vi "re_obj_Datalog Database Info.vi"(0 "method":T9, 1 "initial number (NaN)":dbl=nan format="%.2f", 2 "database {initialize}":path, 5 "tag or base tag":string, 7 "tag config in":T4 {"logging parameters" format="%.2e"; "precision" items=["0", "1", "2", "3", "4", "5", "6", "7", "8", "9", "10", "11", "12", "13", "14", "15", "16", "17"]; "limit delay" format="%.2e"; "deadband" format="%.2e"}, 9 "subsets in":T1[](array[typedef]), 11 "tag index/change#":i32, 12 "meta specifier (not a meta)":T3=enum."not a meta", 13 "initial string (\"\")":string) -> (3 "mode":T2, 4 "tag config list":T4[](array[typedef]) {"logging parameters" format="%.2e"; "precision" items=["0", "1", "2", "3", "4", "5", "6", "7", "8", "9", "10", "11", "12", "13", "14", "15", "16", "17"]; "limit delay" format="%.2e"; "deadband" format="%.2e"}, 6 "#tags/change#":i32, 8 "tag config out":T4 {"logging parameters" format="%.2e"; "precision" items=["0", "1", "2", "3", "4", "5", "6", "7", "8", "9", "10", "11", "12", "13", "14", "15", "16", "17"]; "limit delay" format="%.2e"; "deadband" format="%.2e"}, 10 "subsets out":T1[](array[typedef]), 14 "path":path, 15 "error out":errorcluster)   [LabVIEW 2012]
doc: "Instantiatable object that represents a database through a list of tags and other information. It provides and in-memory copy of the tag info files contained in the tag log directories. These directories are located under the configured data base path.\n\nWhich methods are allowed depends on the mode of the database. When \"locked\" no changes are allowed. When \"unlocked\" everything is allowed. When \"live\" a subset of changes is allowed consistent with ongoing logging.\n\nThe order of the list is kept sorted by tag name. The info cluster holds a seemingly redundant tag index. Its purpose is to allow a list exported via {get list} to be resorted by some other criterion without loosing track of the index.\n\nNote that the handling of the various tag info elements differs. Some are set only when the tag log is first created, some can be set only when the tag is configured before data logging starts, some are determined programatically, and others are modifyable at any time."
uses:
  typedefs/t_DataLog Tag Info List Methods.ctl
  typedefs/t_Datalog Datebase Modes.ctl
  typedefs/clusters/t_DataLog Tag Config.ctl
  typedefs/t_DataLog Temporal Types.ctl
  typedefs/t_DataLog Value Types.ctl
  typedefs/t_DataLog Numerical Format.ctl
  typedefs/t_DataLog Logging Algorithms.ctl
  typedefs/clusters/t_DataLog Tag Subset.ctl
  typedefs/et_DataLog Meta Tag Specifier.ctl
  typedefs/t_Datalog Subsets Actions.ctl
  typedefs/t_DataLog Expression Update Timing Methods.ctl
  subvis/private/glb_DataLog Runtime Parameterisation.vi
  subvis/private/glb_DataLog MCVD.vi
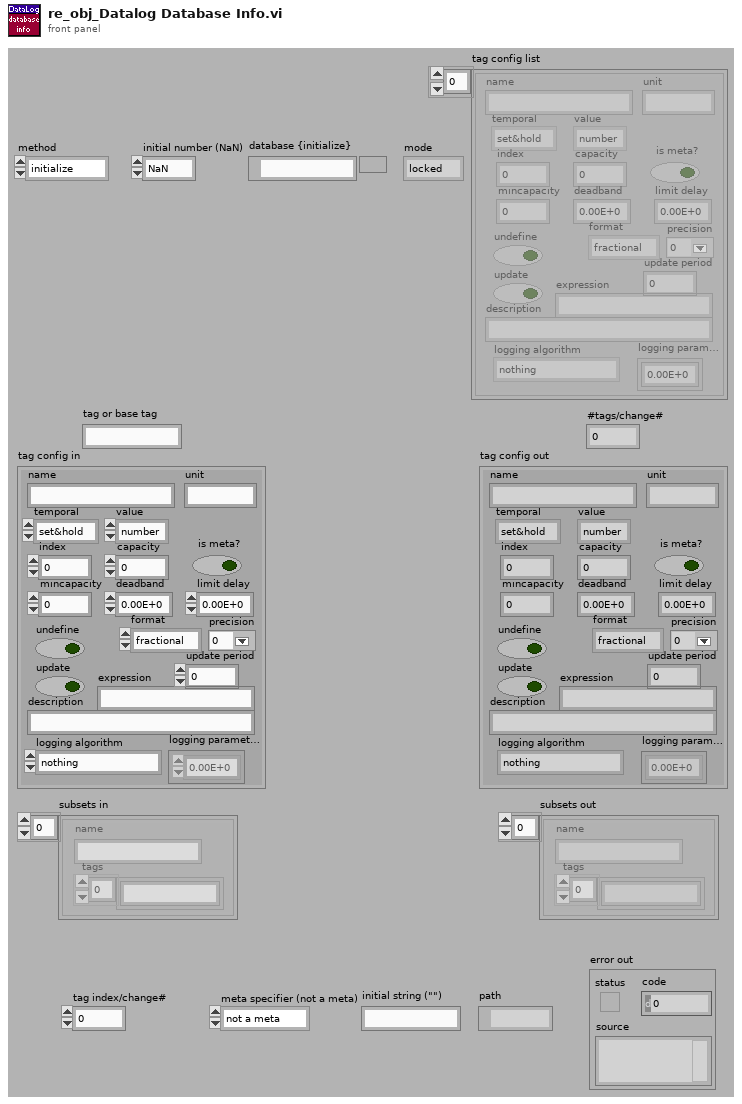
[diagram p1: front panel]
types:
  T1 = typedef "t_DataLog Tag Subset.ctl" = cluster{"name":string, "tags":string[]}
  T2 = typedef "t_Datalog Datebase Modes.ctl" = enum16{"locked", "unlocked", "live", "mirrored"}
  T3 = typedef "et_DataLog Meta Tag Specifier.ctl" = enum32{"warn_lo", "warn_hi", "A_lo", "A_hi", "B_lo", "B_hi", "C_lo", "C_hi", "D_lo", "D_hi", "E_lo", "E_hi", "F_lo", "F_hi", "G_lo", "G_hi", "H_lo", "H_hi", "I_lo", "I_hi", "J_lo", "J_hi", "K_lo", "K_hi", "L_lo", "L_hi", "M_lo", "M_hi", "N_lo", "N_hi", "min", "max", "not a meta"}
  T4 = typedef "t_DataLog Tag Config.ctl" = cluster{"name":string, "unit":string, "temporal":T5, "value":T6, "index":i32, "capacity":i32, "is meta?":bool, "mincapacity":i32, "deadband":dbl, "limit delay":dbl, "format":T7, "precision":u8, "undefine":bool, "update":bool, "update period":u16, "expression":string, "description":string, "logging algorithm":T8, "logging parameters":dbl[]}
  T5 = typedef "t_DataLog Temporal Types.ctl" = enum16{"set&hold", "sample", "event"}
  T6 = typedef "t_DataLog Value Types.ctl" = enum16{"number", "string"}
  T7 = typedef "t_DataLog Numerical Format.ctl" = enum8{"fractional", "exponential", "engineering"}
  T8 = typedef "t_DataLog Logging Algorithms.ctl" = enum16{"nothing", "changes", "everything", "every Nth", "time threshold", "value threshold + prior", "t or v threshold", "t or v threshold + prior"}
  T9 = typedef "t_DataLog Tag Info List Methods.ctl" = enum16{"initialize", "create", "create empty", "rename", "delete", "test tag", "get", "get by name", "get default", "get list", "get path", "get subsets", "set subsets", "set config", "set capacity", "#tags", "go live", "set unlocked", "set mirrored"}
  T10 = typedef "t_Datalog Subsets Actions.ctl" = enum16{"load", "rename", "delete", "save"}
  T11 = typedef "t_DataLog Expression Update Timing Methods.ctl" = enum16{"initialize", "schedule", "make due", "next due", "cleanup"}
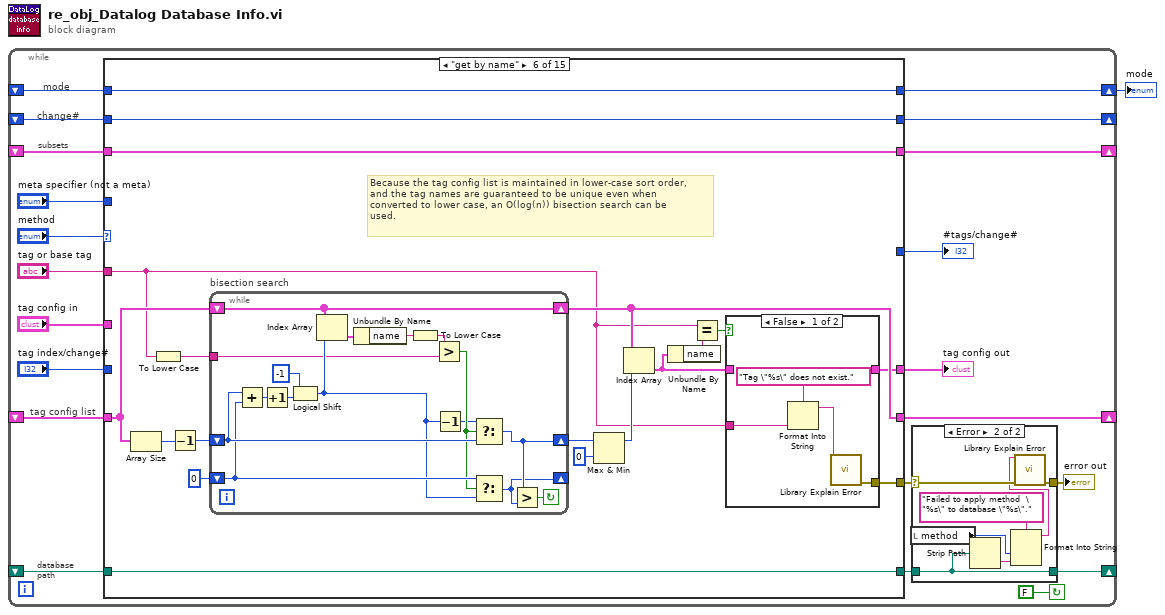
[diagram p0: block diagram]
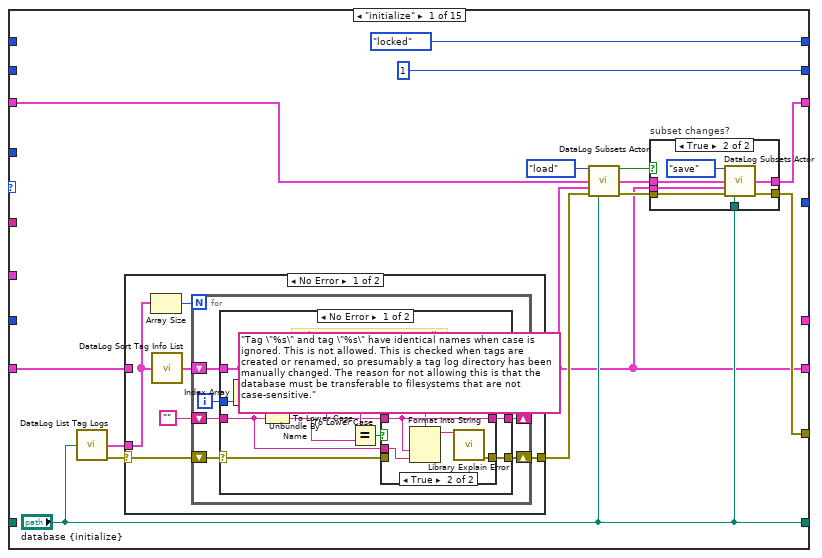
[diagram p3: hidden frame]
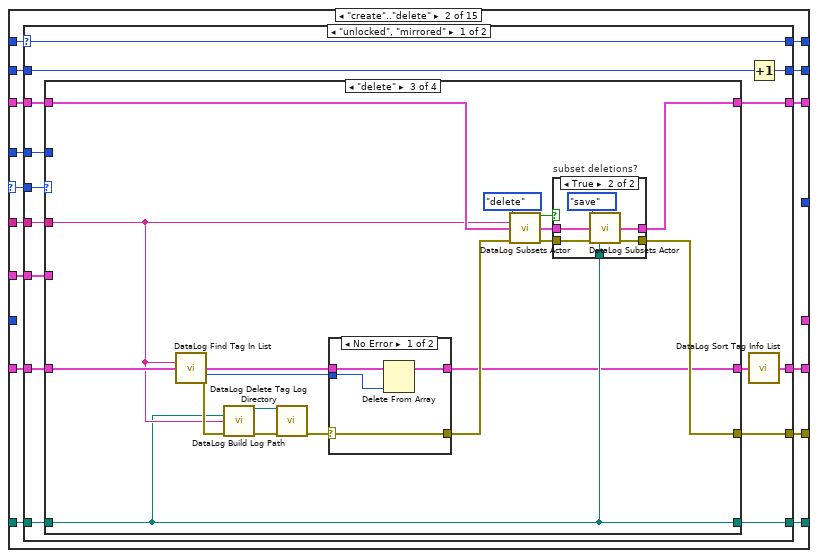
[diagram p8: hidden frame]
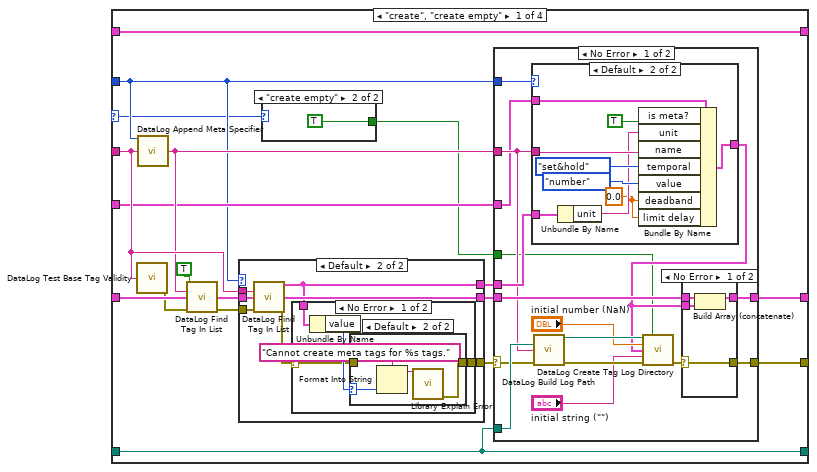
[diagram p9: hidden frame]
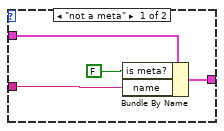
[diagram p11: hidden frame]
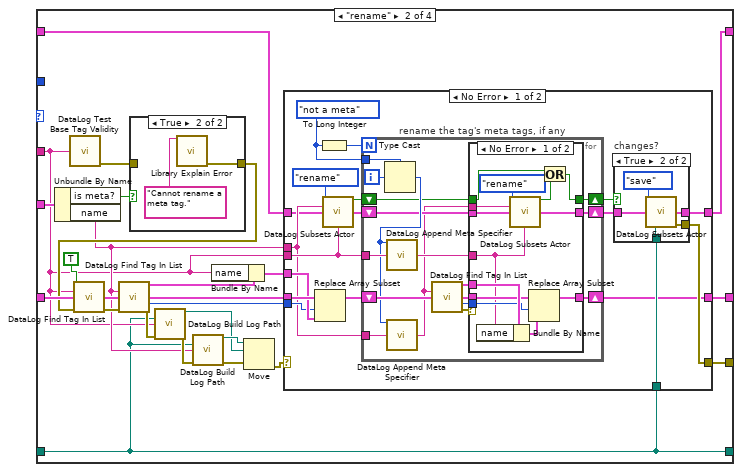
[diagram p17: hidden frame]
diagram:
  n1 = while {
    shift-right: [w21] -> _
    shift-left: _ -> [w20]
    shift-right: [w8] -> w1
    shift-left: _ -> [w18]
    shift-right: [w12] -> _
    shift-left: _ -> [w15]
    shift-right: [w5] -> _
    shift-left: _ -> [w6]
    shift-right: [w3] -> _
    shift-left: _ -> [w4]
    stop <- FALSE continue-if-true
    # "change#"
    # "subsets"
    # "database\npath"
    # "mode"
    # "tag config list"
    n2 = case shown="\"get by name\"" "method" {
      selector: "method" -> [_ w105 w341 _ _ _ _ _ _ _ w465 _ _ _ _]
      tunnel: w20 -> [w44 w104 w340 w364 w373 w384 w421 w439 w454 w458 w473 w589 w595 w601 w607]
      tunnel: [w36 w102 w338 w363 w373 w381 w420 w438 w454 w458 w470 w587 w595 w601 w607] -> w21
      tunnel: "tag config in" -> [_ w101 w337 _ _ _ _ _ _ _ w472 w585 _ _ _]
      tunnel: w18 -> [_ w107 w343 w367 w374 w393 w425 w447 w453 w459 w467 w583 w594 w598 _]
      tunnel: [t_Datalog_Datebase_Modes."locked" ("mode") w106 w342 w367 w374 w393 w425 w447 w453 w459 w466 w583 w594 t_Datalog_Datebase_Modes."unlocked" ("mode") t_Datalog_Datebase_Modes."mirrored" ("mode")] -> w8
      tunnel: [w39 w103 w339 w362 _ w375 w419 _ _ _ w471 _ _ _ _] -> w14
      tunnel: "tag or base tag" -> [_ w100 w336 w361 _ w376 w422 _ _ _ w464 _ _ _ _]
      tunnel: w15 -> [_ w99 w335 w360 w372 w392 w424 w446 w452 w457 w469 w582 w593 w600 w606]
      tunnel: ["database {initialize}" w98 w334 w360 w372 w392 w424 w446 w452 w457 w468 w582 w593 w600 w606] -> w13
      tunnel: [_ _ _ _ w371 w378 w417 _ _ _ _ _ _ _ _] -> w11
      tunnel: "tag index/change#" -> [_ _ _ _ w370 _ _ w444 _ _ _ w581 _ _ _]
      tunnel: "meta specifier (not a meta)" -> [_ w97 w333 _ _ _ _ _ _ _ _ _ _ _ _]
      tunnel: [w34 w95 w331 w359 w369 w391 w416 w445 w451 w456 w462 w580 w592 w597 w604] -> w5
      tunnel: w6 -> [w41 w96 w332 w359 w369 w391 w416 w445 w451 w456 w463 w580 w592 w597 w604]
      tunnel: w4 -> [_ w94 w330 w358 w368 w390 w415 w440 w450 w455 w461 w579 w590 w596 w603]
      tunnel: [1 w93 w329 w358 w368 w390 w415 w440 w450 w455 w460 w578 w590 w596 w603] -> w3
      tunnel: [_ _ _ _ _ _ _ w440 _ _ _ _ w591 _ _] -> w2
      frame "initialize" {
        n3 = call "DataLog List Tag Logs.vi"("database path"="database {initialize}") -> ("tag info list"=w45:T4[], "error out"=w46:errorcluster)  [unwired: 13 in]
        n4 = case shown="No Error" w46 {
          selector: w46 -> [w61 w92]
          tunnel: [w60 w92] -> w40
          tunnel: [w59 w91] -> w36
          tunnel: w45 -> [w56 _]
          tunnel: w44 -> [_ w91]
          frame No Error {
            n5 = Array Size(array=w56) -> (size(s)=w57:i32)
            n6 = call "DataLog Sort Tag Info List.vi"("tag list in"=w56) -> ("tag list out"=w62:T4[])  [unwired: 14 in]
            n7 = for {
              N: w57 -> [_]
              shift-right: [w65] -> w60
              shift-left: w61 -> [w67]
              shift-right: [w66] -> w59
              shift-left: w62 -> [w69]
              shift-right: [w64] -> _
              shift-left: "" -> [w63]
              i -> [w68]
              n8 = case shown="No Error" w67 {
                selector: w67 -> [w74 w89]
                tunnel: w69 -> [w79 w90]
                tunnel: w68 -> [w80 _]
                tunnel: [w79 w90] -> w66
                tunnel: [w73 w89] -> w65
                tunnel: [w71 w88] -> w64
                tunnel: w63 -> [w70 w88]
                frame No Error {
                  # "Make sure tag names are still\ncase-independently unique."
                  n9 = Index Array(array=w79, index=w80) -> (element=w78:T4)
                  n10 = To Lower Case(string=w70) -> (all lower case string=w76:string)
                  n11 = Unbundle By Name(w78) -> ("name"=w72:string)
                  n12 = To Lower Case(string=w72) -> (all lower case string=w77:string)
                  n13 = Equal?(x=w77, y=w76) -> (x = y?=w75:bool)
                  n14 = case shown="True" w75 {
                    tunnel: w74 -> [w82 _]
                    tunnel: [w82 w87] -> w73
                    tunnel: w72 -> [w81 w85]
                    tunnel: [w81 w85] -> w71
                    tunnel: w70 -> [_ w84]
                    frame False {
                    }
                    frame True {
                      n15 = Format Into String(format string="Tag \"%s\" and tag \"%s\" have identical names when case is ignored. This is not allowed. This is checked when tags are created or renamed, so presumably a tag log directory has been manually changed. The reason for not allowing this is that the database must be transferable to filesystems that are not case-sensitive.", w85, w84) -> (resulting string=w86:string)  [unwired: 2 in, 1 out]
                      n16 = call "Library Explain Error.vi"("explanation prefix (none)"=w86) -> ("explained error"=w87:errorcluster)  [unwired: 14 in]
                    }
                  }
                }
                frame Error {
                }
              }
            }
          }
          frame Error {
          }
        }
        n17 = call "DataLog Subsets Actor.vi"("action"=t_Datalog_Subsets_Actions."load", "subsets in"=w41, "tag config list"=w36, "error in (no error)"=w40, "database path"="database {initialize}") -> ("changes"=w33:bool, "subset out"=w35:T1[], "error out"=w38:errorcluster)  [unwired: 8 in]
        n18 = case "subset changes?" shown="True" w33 {
          tunnel: [w47 w54] -> w39
          tunnel: w38 -> [w47 w53]
          tunnel: "database {initialize}" -> [_ w52]
          tunnel: w36 -> [_ w51]
          tunnel: w35 -> [w48 w50]
          tunnel: [w48 w49] -> w34
          frame False {
          }
          frame True {
            n19 = call "DataLog Subsets Actor.vi"("action"=t_Datalog_Subsets_Actions."save", "subsets in"=w50, "tag config list"=w51, "error in (no error)"=w53, "database path"=w52) -> ("subset out"=w49:T1[], "error out"=w54:errorcluster)  [unwired: 8 in, 1 out]
          }
        }
      }
      frame "create".."delete" {
        n20 = case shown="\"unlocked\", \"mirrored\"" w107 {
          selector: w107 -> [w109 w324]
          tunnel: [w109 w324] -> w106
          tunnel: w105 -> [w122 _]
          tunnel: w104 -> [w121 w325]
          tunnel: [w118 w328] -> w103
          tunnel: [w116 w325] -> w102
          tunnel: w101 -> [w119 _]
          tunnel: w100 -> [w120 _]
          tunnel: w99 -> [w115 w323]
          tunnel: [w113 w323] -> w98
          tunnel: w97 -> [w114 _]
          tunnel: w96 -> [w112 w322]
          tunnel: [w111 w322] -> w95
          tunnel: w94 -> [w110 w321]
          tunnel: [w108 w321] -> w93
          frame "unlocked", "mirrored" {
            n21 = case shown="\"delete\"" w122 {
              selector: w122 -> [w124 _ _ _]
              tunnel: w121 -> [w140 w209 w301 w320]
              tunnel: [w136 w204 w286 w320] -> w117
              tunnel: w120 -> [w134 w199 w294 _]
              tunnel: w119 -> [w129 w222 _ _]
              tunnel: [w137 w200 w289 _] -> w118
              tunnel: w115 -> [w126 w198 w287 w319]
              tunnel: w114 -> [w128 _ _ _]
              tunnel: [w126 w198 w287 w319] -> w113
              tunnel: w112 -> [w125 w203 w295 w318]
              tunnel: [w125 w202 w291 w318] -> w111
              frame "create", "create empty" {
                n22 = call "DataLog Test Base Tag Validity.vi"("base tag"=w134) -> ("error out"=w138:errorcluster)  [unwired: 13 in, 1 out]
                n23 = call "DataLog Append Meta Specifier.vi"("meta specifier"=w128, "tag in"=w134) -> ("tag out"=w130:string)  [unwired: 13 in]
                n24 = call "DataLog Find Tag In List.vi"("may not exist (false)"=TRUE, "tag"=w130, "tag config list in"=w140, "error in (no error)"=w138) -> ("tag config list out"=w131:T4[], "error out"=w135:errorcluster)  [unwired: 8 in, 2 out]
                n25 = case shown="Default" w128 {
                  tunnel: w135 -> [w179 w187]
                  tunnel: [w179 w181] -> w127
                  tunnel: w134 -> [_ w186]
                  tunnel: w131 -> [w180 w185]
                  tunnel: [w180 w184] -> w133
                  tunnel: [_ w183] -> w132
                  frame "not a meta" {
                  }
                  frame Default {
                    n26 = call "DataLog Find Tag In List.vi"("tag"=w186, "tag config list in"=w185, "error in (no error)"=w187) -> ("tag config out"=w183:T4, "tag config list out"=w184:T4[], "error out"=w182:errorcluster)  [unwired: 9 in, 1 out]
                    n27 = case shown="No Error" w182 {
                      selector: w182 -> [w189 w197]
                      tunnel: w183 -> [w191 _]
                      tunnel: [w188 w197] -> w181
                      frame No Error {
                        n28 = Unbundle By Name(w191) -> ("value"=w190:T6)
                        n29 = case shown="Default" w190 {
                          selector: w190 -> [_ w194]
                          tunnel: w189 -> [w192 _]
                          tunnel: [w192 w196] -> w188
                          frame "number" {
                          }
                          frame Default {
                            n30 = Format Into String(format string="Cannot create meta tags for %s tags.", w194) -> (resulting string=w195:string)  [unwired: 2 in, 1 out]
                            n31 = call "Library Explain Error.vi"("explanation prefix (none)"=w195) -> ("explained error"=w196:errorcluster)  [unwired: 14 in]
                          }
                        }
                      }
                      frame Error {
                      }
                    }
                  }
                }
                n32 = case shown="\"create empty\"" w124 {
                  tunnel: [_ TRUE] -> w123
                  frame Default {
                  }
                  frame "create empty" {
                  }
                }
                n33 = case shown="No Error" w127 {
                  selector: w127 -> [w144 w177]
                  tunnel: [w154 w177] -> w137
                  tunnel: [w153 w178] -> w136
                  tunnel: w133 -> [w151 w178]
                  tunnel: w132 -> [w150 _]
                  tunnel: w126 -> [w149 _]
                  tunnel: w130 -> [w147 _]
                  tunnel: w129 -> [w146 _]
                  tunnel: w128 -> [w145 _]
                  tunnel: w123 -> [w142 _]
                  frame No Error {
                    n34 = case shown="Default" w145 {
                      tunnel: w147 -> [w160 w170]
                      tunnel: w150 -> [_ w166]
                      tunnel: [w159 w164] -> w148
                      tunnel: w146 -> [w158 w163]
                      frame "not a meta" {
                        n35 = Bundle By Name(cluster=w158, "is meta?"=FALSE, "name"=w160) -> (w159:T4)
                      }
                      frame Default {
                        w162 = 0.0 ("deadband")
                        n36 = Unbundle By Name(w166) -> ("unit"=w165:string)
                        n37 = Bundle By Name(cluster=w163, "is meta?"=TRUE, "unit"=w165, "name"=w170, "temporal"=t_DataLog_Temporal_Types."set&hold", "value"=t_DataLog_Value_Types."number" ("valuation"), "deadband"=w162, "limit delay"=w162) -> (w164:T4)
                      }
                    }
                    n38 = call "DataLog Build Log Path.vi"("database path"=w149, "tag"=w147, "error in (no error)"=w144) -> ("tag log directory"=w156:path, "error out"=w157:errorcluster)  [unwired: 11 in]
                    n39 = call "DataLog Create Tag Log Directory.vi"("tag log directory"=w156, "no initial? (false)"=w142, "initial number (NaN)"="initial number (NaN)", "initial tag config"=w148, "initial string (\"\")"="initial string (\"\")", "error in (no error)"=w157) -> ("error out"=w155:errorcluster)  [unwired: 8 in, 1 out]
                    n40 = case shown="No Error" w155 {
                      selector: w155 -> [w171 w176]
                      tunnel: [w171 w176] -> w154
                      tunnel: [w173 w175] -> w153
                      tunnel: w151 -> [w174 w175]
                      tunnel: w148 -> [w172 _]
                      frame No Error {
                        n41 = Build Array (concatenate)(w174, w172) -> (w173:T4[])
                      }
                      frame Error {
                      }
                    }
                  }
                  frame Error {
                  }
                }
              }
              frame "rename" {
                n42 = Unbundle By Name(w222) -> ("is meta?"=w221:bool, "name"=w201:string)
                n43 = call "DataLog Test Base Tag Validity.vi"("base tag"=w199) -> ("error out"=w211:errorcluster)  [unwired: 13 in, 1 out]
                n44 = case shown="True" w221 {
                  tunnel: w211 -> [w283 _]
                  tunnel: [w283 w285] -> w206
                  frame False {
                  }
                  frame True {
                    n45 = call "Library Explain Error.vi"("explanation prefix (none)"="Cannot rename a meta tag.") -> ("explained error"=w285:errorcluster)  [unwired: 14 in]
                  }
                }
                n46 = call "DataLog Find Tag In List.vi"("may not exist (false)"=TRUE, "tag"=w199, "tag config list in"=w209, "error in (no error)"=w206) -> ("tag config list out"=w208:T4[], "error out"=w207:errorcluster)  [unwired: 8 in, 2 out]
                n47 = call "DataLog Find Tag In List.vi"("tag"=w201, "tag config list in"=w208, "error in (no error)"=w207) -> ("tag config out"=w212:T4, "tag config list out"=w213:T4[], "tag index"=w214:i32, "error out"=w210:errorcluster)  [unwired: 9 in]
                n48 = call "DataLog Build Log Path.vi"("database path"=w198, "tag"=w199, "error in (no error)"=w210) -> ("tag log directory"=w217:path, "error out"=w219:errorcluster)  [unwired: 11 in]
                n49 = call "DataLog Build Log Path.vi"("database path"=w198, "tag"=w201, "error in (no error)"=w219) -> ("tag log directory"=w220:path, "error out"=w218:errorcluster)  [unwired: 11 in]
                n50 = Bundle By Name(cluster=w212, "name"=w199) -> (w215:T4)
                n51 = Move(source path=w220, error in=w218, 10:w217) -> (error out=w216:errorcluster)  [unwired: 2 in, 2 out]
                n52 = case shown="No Error" w216 {
                  selector: w216 -> [_ w282]
                  tunnel: [w229 w282] -> w200
                  tunnel: w213 -> [w240 w281]
                  tunnel: [w224 w281] -> w204
                  tunnel: w215 -> [w239 _]
                  tunnel: w214 -> [w238 _]
                  tunnel: w203 -> [w223 w280]
                  tunnel: [w227 w280] -> w202
                  tunnel: w201 -> [w231 _]
                  tunnel: w199 -> [w232 _]
                  tunnel: w198 -> [w226 _]
                  frame No Error {
                    w235 = et_DataLog_Meta_Tag_Specifier."not a meta" ("limit specifier")
                    n53 = Replace Array Subset(array=w240, new element=w239, index=w238) -> (w236:T4[])
                    n54 = To Long Integer(number=w235) -> (32bit integer=w237:i32)
                    n55 = call "DataLog Subsets Actor.vi"("action"=t_Datalog_Subsets_Actions."rename", "tag"=w231, "subsets in"=w223, "new name"=w232) -> ("changes"=w230:bool, "subset out"=w233:T1[])  [unwired: 9 in, 1 out]
                    n56 = for "rename the tag's meta tags, if any" {
                      N: w237 -> [_]
                      shift-right: [w254] -> w224
                      shift-left: w236 -> [w261]
                      tunnel: w235 -> [w263]
                      tunnel: w231 -> [w260]
                      tunnel: w232 -> [w259]
                      shift-right: [w250] -> w228
                      shift-left: w233 -> [w251]
                      shift-right: [w247] -> w225
                      shift-left: w230 -> [w248]
                      i -> [w262]
                      n57 = Type Cast(type=w263, x=w262) -> (*(type *) &x=w252:T3)
                      n58 = call "DataLog Append Meta Specifier.vi"("meta specifier"=w252, "tag in"=w259) -> ("tag out"=w257:string)  [unwired: 13 in]
                      n59 = call "DataLog Append Meta Specifier.vi"("meta specifier"=w252, "tag in"=w260) -> ("tag out"=w249:string)  [unwired: 13 in]
                      n60 = call "DataLog Find Tag In List.vi"("tag"=w249, "tag config list in"=w261) -> ("tag config out"=w258:T4, "tag config list out"=w255:T4[], "tag index"=w253:i32, "error out"=w256:errorcluster)  [unwired: 10 in]
                      n61 = case shown="No Error" w256 {
                        tunnel: w258 -> [w276 _]
                        tunnel: w257 -> [w267 _]
                        tunnel: w255 -> [w275 w279]
                        tunnel: [w274 w279] -> w254
                        tunnel: w253 -> [w273 _]
                        tunnel: w251 -> [w270 w278]
                        tunnel: [w269 w278] -> w250
                        tunnel: w249 -> [w268 _]
                        tunnel: w248 -> [w266 w277]
                        tunnel: [w264 w277] -> w247
                        frame No Error {
                          n62 = Bundle By Name(cluster=w276, "name"=w267) -> (w272:T4)
                          n63 = call "DataLog Subsets Actor.vi"("action"=t_Datalog_Subsets_Actions."rename", "tag"=w268, "subsets in"=w270, "new name"=w267) -> ("changes"=w265:bool, "subset out"=w269:T1[])  [unwired: 9 in, 1 out]
                          n64 = Replace Array Subset(array=w275, new element=w272, index=w273) -> (w274:T4[])
                          n65 = Or(x=w266, y=w265) -> (x .or. y?=w264:bool)
                        }
                        frame Error {
                        }
                      }
                    }
                    n66 = case "changes?" shown="True" w225 {
                      tunnel: w228 -> [w241 w245]
                      tunnel: [w241 w244] -> w227
                      tunnel: [_ w243] -> w229
                      tunnel: w226 -> [_ w242]
                      frame False {
                      }
                      frame True {
                        n67 = call "DataLog Subsets Actor.vi"("action"=t_Datalog_Subsets_Actions."save", "subsets in"=w245, "database path"=w242) -> ("subset out"=w244:T1[], "error out"=w243:errorcluster)  [unwired: 10 in, 1 out]
                      }
                    }
                  }
                  frame Error {
                  }
                }
              }
              frame "delete" {
                n68 = call "DataLog Find Tag In List.vi"("tag"=w294, "tag config list in"=w301) -> ("tag config list out"=w298:T4[], "tag index"=w299:i32, "error out"=w300:errorcluster)  [unwired: 10 in, 1 out]
                n69 = call "DataLog Build Log Path.vi"("database path"=w287, "tag"=w294, "error in (no error)"=w300) -> ("tag log directory"=w303:path, "error out"=w302:errorcluster)  [unwired: 11 in]
                n70 = call "DataLog Delete Tag Log Directory.vi"("tag log directory"=w303, "error in (no error)"=w302) -> ("error out"=w297:errorcluster)  [unwired: 12 in, 1 out]
                n71 = case shown="No Error" w297 {
                  selector: w297 -> [w312 w316]
                  tunnel: [w315 w317] -> w286
                  tunnel: w299 -> [w314 _]
                  tunnel: w298 -> [w313 w317]
                  tunnel: [w312 w316] -> w296
                  frame No Error {
                    n72 = Delete From Array(array=w313, index=w314) -> (array with subset deleted=w315:T4[])  [unwired: 1 in, 1 out]
                  }
                  frame Error {
                  }
                }
                n73 = call "DataLog Subsets Actor.vi"("action"=t_Datalog_Subsets_Actions."delete", "tag"=w294, "subsets in"=w295, "error in (no error)"=w296) -> ("changes"=w288:bool, "subset out"=w292:T1[], "error out"=w290:errorcluster)  [unwired: 9 in]
                n74 = case "subset deletions?" shown="True" w288 {
                  tunnel: w292 -> [w305 w310]
                  tunnel: [w305 w309] -> w291
                  tunnel: w290 -> [w304 w308]
                  tunnel: [w304 w307] -> w289
                  tunnel: w287 -> [_ w306]
                  frame False {
                  }
                  frame True {
                    n75 = call "DataLog Subsets Actor.vi"("action"=t_Datalog_Subsets_Actions."save", "subsets in"=w310, "error in (no error)"=w308, "database path"=w306) -> ("subset out"=w309:T1[], "error out"=w307:errorcluster)  [unwired: 9 in, 1 out]
                  }
                }
              }
              frame Default {
                # "should never happen"
              }
            }
            n76 = Increment(x=w110) -> (x+1=w108:i32)
            n77 = call "DataLog Sort Tag Info List.vi"("tag list in"=w117) -> ("tag list out"=w116:T4[])  [unwired: 14 in]
          }
          frame "locked", "live" {
            n78 = Format Into String(format string="Operation not allowed while the database is %s.", w324) -> (resulting string=w327:string)  [unwired: 2 in, 1 out]
            n79 = call "Library Explain Error.vi"("explanation prefix (none)"=w327) -> ("explained error"=w328:errorcluster)  [unwired: 14 in]
          }
        }
      }
      frame "go live" {
        n80 = case shown="\"locked\", \"live\", \"mirrored\"" w343 {
          selector: w343 -> [_ w353]
          tunnel: [t_Datalog_Datebase_Modes."live" ("mode") w353] -> w342
          tunnel: w341 -> [_ _]
          tunnel: w340 -> [w344 w354]
          tunnel: [_ w357] -> w339
          tunnel: [w344 w354] -> w338
          tunnel: w337 -> [_ _]
          tunnel: w336 -> [_ _]
          tunnel: w335 -> [w348 w352]
          tunnel: [w348 w352] -> w334
          tunnel: w333 -> [_ _]
          tunnel: w332 -> [w347 w351]
          tunnel: [w347 w351] -> w331
          tunnel: w330 -> [w346 w350]
          tunnel: [w346 w350] -> w329
          frame "unlocked" {
            n81 = Array Size(array=w344) -> (size(s)=w345:i32)
            n82 = global write "glb_DataLog Runtime Parameterisation.vi" "#tags"(w345) -> ()
          }
          frame "locked", "live", "mirrored" {
            n83 = Format Into String(format string="Operation not allowed while the database is %s.", w353) -> (resulting string=w356:string)  [unwired: 2 in, 1 out]
            n84 = call "Library Explain Error.vi"("explanation prefix (none)"=w356) -> ("explained error"=w357:errorcluster)  [unwired: 14 in]
          }
        }
      }
      frame "test tag" {
        # "Expose these preliminary checks through this object method so as to make them available for remote calling."
        n85 = call "DataLog Test Base Tag Validity.vi"("base tag"=w361) -> ("error out"=w365:errorcluster)  [unwired: 13 in, 1 out]
        n86 = call "DataLog Find Tag In List.vi"("may not exist (false)"=TRUE, "tag"=w361, "tag config list in"=w364, "error in (no error)"=w365) -> ("tag config list out"=w363:T4[], "error out"=w362:errorcluster)  [unwired: 8 in, 2 out]
      }
      frame "get" {
        n87 = Index Array(array=w373, index=w370) -> (element=w371:T4)
      }
      frame "get by name" {
        # "Because the tag config list is maintained in lower-case sort order,\nand the tag names are guaranteed to be unique even when\nconverted to lower case, an O(log(n)) bisection search can be\nused."
        n88 = Array Size(array=w384) -> (size(s)=w385:i32)
        n89 = To Lower Case(string=w376) -> (all lower case string=w383:string)
        n90 = Decrement(x=w385) -> (x-1=w389:i32)
        n91 = while "bisection search" {
          shift-right: [w406] -> _
          shift-left: 0 -> [w413]
          shift-right: [w412] -> w387
          shift-left: w389 -> [w414]
          tunnel: w383 -> [w403]
          shift-right: [w401] -> w381
          shift-left: w384 -> [w401]
          stop <- w411 continue-if-true
          n92 = Add(x=w414, y=w413) -> (x+y=w409:i32)
          n93 = Increment(x=w409) -> (x+1=w404:i32)
          n94 = Logical Shift(y=-1, x=w404) -> (x << y=w407:i32)
          n95 = Index Array(array=w401, index=w407) -> (element=w402:T4)
          n96 = Unbundle By Name(w402) -> ("name"=w400:string)
          n97 = To Lower Case(string=w400) -> (all lower case string=w399:string)
          n98 = Greater?(x=w399, y=w403) -> (0:w410:bool)
          n99 = Decrement(x=w407) -> (x-1=w405:i32)
          n100 = Select(t=w405, s=w410, f=w414) -> (s? t:f=w412:i32)
          n101 = Select(t=w413, s=w410, f=w407) -> (s? t:f=w406:i32)
          n102 = Greater?(x=w412, y=w406) -> (0:w411:bool)
        }
        n103 = Max & Min(x=w387, y=0) -> (max(x,y)=w382:i32)  [unwired: 1 out]
        n104 = Index Array(array=w381, index=w382) -> (element=w377:T4)
        n105 = Unbundle By Name(w377) -> ("name"=w380:string)
        n106 = Equal?(x=w376, y=w380) -> (x = y?=w379:bool)
        n107 = case shown="False" w379 {
          tunnel: w377 -> [_ w398]
          tunnel: [_ w398] -> w378
          tunnel: w376 -> [w396 _]
          tunnel: [w395 _] -> w375
          frame False {
            n108 = Format Into String(format string="Tag \"%s\" does not exist.", w396) -> (resulting string=w394:string)  [unwired: 2 in, 1 out]
            n109 = call "Library Explain Error.vi"("explanation prefix (none)"=w394) -> ("explained error"=w395:errorcluster)  [unwired: 14 in]
          }
          frame True {
          }
        }
      }
      frame "get default" {
        n110 = global read "glb_DataLog MCVD.vi" "default config"() -> (w418:T4)
        n111 = Empty String/Path?(string/path=w422) -> (empty?=w423:bool)
        n112 = case "no base tag specified?" shown="False" w423 {
          tunnel: w421 -> [w435 w437]
          tunnel: w422 -> [w434 _]
          tunnel: [w433 w437] -> w420
          tunnel: [w431 _] -> w419
          tunnel: w418 -> [w429 w436]
          tunnel: [w426 w436] -> w417
          frame False {
            n113 = call "DataLog Find Tag In List.vi"("tag"=w434, "tag config list in"=w435) -> ("tag config out"=w432:T4, "tag config list out"=w433:T4[], "error out"=w431:errorcluster)  [unwired: 10 in, 1 out]
            n114 = Unbundle By Name(w432) -> ("format"=w430:T7, "precision"=w427:u8)
            n115 = Bundle By Name(cluster=w429, "format"=w430, "precision"=w427, "logging algorithm"=t_DataLog_Logging_Algorithms."everything" ("default logging algorithm")) -> (w426:T4)
          }
          frame True {
          }
        }
      }
      frame "get list" {
        # "By only returning the list when the change# is\ndifferent (or has not been wired) the caller can\nprevent getting the same list twice.\n\nThough the prevention is not 100% because\na failed update sometimes bumps the change\ncount and, after 2^32 updates, the count\nwraps to 0, it prevents the vast majority of\nsuperfluous list fetches. This is of importance\nwhen polling the list over the network."
        n116 = Not Equal?(x=w440, y=w444) -> (x != y?=w443:bool)
        n117 = Equal To 0?(x=w444) -> (x = 0?=w442:bool)
        n118 = Or(x=w443, y=w442) -> (x .or. y?=w441:bool)
        n119 = case shown="True" w441 {
          tunnel: w439 -> [w448 w449]
          tunnel: [w448 w449] -> w438
          frame False {
          }
          frame True {
            "tag config list" <- w449
          }
        }
      }
      frame "get path" {
        "path" <- w452
      }
      frame "get subsets" {
        "subsets out" <- w456
      }
      frame "set subsets", "set config" {
        n120 = case shown="\"unlocked\"..\"mirrored\"" w467 {
          selector: w467 -> [w478 w489]
          tunnel: w473 -> [w481 w493]
          tunnel: w472 -> [_ w492]
          tunnel: [w477 w491] -> w471
          tunnel: [w481 w490] -> w470
          tunnel: w469 -> [w476 w484]
          tunnel: [w476 w484] -> w468
          tunnel: [w478 w489] -> w466
          tunnel: w465 -> [_ w487]
          tunnel: w464 -> [_ w488]
          tunnel: w463 -> [w475 w486]
          tunnel: [w475 w485] -> w462
          tunnel: w461 -> [w474 w483]
          tunnel: [w474 w482] -> w460
          frame "locked" {
            n121 = Format Into String(format string="Operation not allowed while the database is %s.", w478) -> (resulting string=w480:string)  [unwired: 2 in, 1 out]
            n122 = call "Library Explain Error.vi"("explanation prefix (none)"=w480) -> ("explained error"=w477:errorcluster)  [unwired: 14 in]
          }
          frame "unlocked".."mirrored" {
            n123 = case shown="\"set config\"" w487 {
              tunnel: w493 -> [w496 w514 w576]
              tunnel: w492 -> [_ w509 _]
              tunnel: [w498 w508 _] -> w491
              tunnel: [w496 w507 w576] -> w490
              tunnel: w484 -> [w497 w506 _]
              tunnel: w488 -> [_ w505 _]
              tunnel: w486 -> [_ w504 w577]
              tunnel: [w500 w504 w577] -> w485
              tunnel: w483 -> [w495 w502 w575]
              tunnel: [w494 w503 w575] -> w482
              frame "set subsets" {
                n124 = call "DataLog Subsets Actor.vi"("action"=t_Datalog_Subsets_Actions."save", "subsets in"="subsets in", "database path"=w497) -> ("subset out"=w500:T1[], "error out"=w498:errorcluster)  [unwired: 10 in, 1 out]
                n125 = Increment(x=w495) -> (x+1=w494:i32)
              }
              frame "set config" {
                n126 = call "DataLog Find Tag In List.vi"("tag"=w505, "tag config list in"=w514) -> ("tag config out"=w513:T4, "tag config list out"=w512:T4[], "tag index"=w510:i32, "error out"=w511:errorcluster)  [unwired: 10 in]
                n127 = case shown="No Error" w511 {
                  selector: w511 -> [_ w574]
                  tunnel: w513 -> [w528 _]
                  tunnel: w512 -> [w539 w573]
                  tunnel: w510 -> [w538 _]
                  tunnel: w509 -> [w523 _]
                  tunnel: [w530 w574] -> w508
                  tunnel: [w532 w573] -> w507
                  tunnel: w505 -> [w531 _]
                  tunnel: w506 -> [w518 _]
                  tunnel: w502 -> [w516 w572]
                  tunnel: [w515 w572] -> w503
                  frame No Error {
                    # "Preserve the tag info elements that\nare not allowed to change at run time."
                    n128 = Unbundle By Name(w528) -> ("update"=w521:bool, "name"=w533:string, "unit"=w534:string, "temporal"=w535:T5, "value"=w536:T6, "index"=w537:i32, "capacity"=w529:i32, "is meta?"=w517:bool)
                    n129 = Unbundle By Name(w523) -> ("update"=w522:bool)
                    n130 = Or(x=w522, y=w521) -> (x .or. y?=w520:bool)
                    n131 = case shown="True" w517 {
                      selector: w517 -> [w541 w550]
                      tunnel: w537 -> [w549 w558]
                      tunnel: w536 -> [w548 w557]
                      tunnel: w535 -> [w547 w556]
                      tunnel: w534 -> [w546 w555]
                      tunnel: w533 -> [w545 w554]
                      tunnel: w529 -> [w544 w553]
                      tunnel: [w543 w552] -> w525
                      tunnel: w523 -> [w542 w551]
                      frame True {
                        w540 = 0.0 ("deadband")
                        n132 = Bundle By Name(cluster=w542, "name"=w545, "unit"=w546, "temporal"=w547, "value"=w548, "index"=w549, "capacity"=w544, "is meta?"=w541, "deadband"=w540, "limit delay"=w540) -> (w543:T4)
                      }
                      frame False {
                        n133 = Bundle By Name(cluster=w551, "name"=w554, "unit"=w555, "temporal"=w556, "value"=w557, "index"=w558, "capacity"=w553, "is meta?"=w550) -> (w552:T4)
                      }
                    }
                    n134 = call "DataLog Build Log Path.vi"("database path"=w518, "tag"=w531) -> ("tag log directory"=w526:path, "error out"=w524:errorcluster)  [unwired: 12 in]
                    n135 = call "DataLog Save or Load Tag Config.vi"("tag log directory"=w526, "action"=enum16{"save", "load"}."save", "tag config in"=w525, "error in (no error)"=w524) -> ("error out"=w527:errorcluster)  [unwired: 9 in, 2 out]
                    n136 = case shown="No Error" w527 {
                      selector: w527 -> [w564 w571]
                      tunnel: w539 -> [w566 w570]
                      tunnel: w538 -> [w561 _]
                      tunnel: [w565 w570] -> w532
                      tunnel: w525 -> [w563 _]
                      tunnel: [w564 w571] -> w530
                      tunnel: w520 -> [w562 _]
                      tunnel: [w559 w569] -> w515
                      tunnel: w516 -> [w560 w569]
                      frame No Error {
                        n137 = case shown="True" w562 {
                          tunnel: w561 -> [_ w567]
                          frame False {
                          }
                          frame True {
                            n138 = call "obj_DataLog Expression Update Timing.vi"("method"=t_DataLog_Expression_Update_Timing_Methods."make due", "tag index"=w567) -> ()  [unwired: 12 in, 2 out]
                          }
                        }
                        n139 = Increment(x=w560) -> (x+1=w559:i32)
                        n140 = Replace Array Subset(array=w566, new element=w563, index=w561) -> (w565:T4[])
                      }
                      frame Error {
                      }
                    }
                  }
                  frame Error {
                  }
                }
              }
              frame Default {
                # "should never happen"
              }
            }
          }
        }
      }
      frame "set capacity" {
        n141 = Unbundle By Name(w585) -> ("capacity"=w584:i32)
        n142 = Index Array(array=w589, index=w581) -> (element=w588:T4)
        n143 = Increment(x=w579) -> (x+1=w578:i32)
        n144 = Bundle By Name(cluster=w588, "capacity"=w584) -> (w586:T4)
        n145 = Replace Array Subset(array=w589, new element=w586, index=w581) -> (w587:T4[])
      }
      frame "#tags" {
        n146 = Array Size(array=w595) -> (size(s)=w591:i32)
      }
      frame "set unlocked" {
        n147 = case shown="\"live\"" w598 {
          frame Default {
          }
          frame "live" {
            n148 = global write "glb_DataLog Runtime Parameterisation.vi" "#tags"(0 ("#tags")) -> ()
          }
        }
      }
      frame "set mirrored" {
      }
    }
    "tag config out" <- w11
    "#tags/change#" <- w2
    n149 = case shown="Error" w14 {
      selector: w14 -> [w24 w31]
      tunnel: w13 -> [w23 w25]
      tunnel: [w23 w25] -> w12
      tunnel: [w24 w30] -> w7
      frame No Error {
      }
      frame Error {
        n150 = local read "method"() -> (w29:T9)
        n151 = Strip Path(path=w25) -> (name=w26:string)  [unwired: 1 out]
        n152 = Format Into String(format string="Failed to apply method  \"%s\" to database \"%s\".", w29, w26) -> (resulting string=w27:string)  [unwired: 2 in, 1 out]
        n153 = call "Library Explain Error.vi"("explanation prefix (none)"=w27, "error in (no error)"=w31) -> ("explained error"=w30:errorcluster)  [unwired: 13 in]
      }
    }
    "error out" <- w7
  }
  "mode" <- w1
